vi "SEK2020v1SubVIAndarReto.vi"(1 "NXT/EV3":T1) -> (8 "NXT/EV3 2":T1)   [LabVIEW 2016]
uses:
  <vilib>/NXT/Subs/LVHSConnector.ctl
  <vilib>/NXT/LegoClasses/BrickReference/BrickReference.lvclass
  <vilib>/NXT/Block Support/NXT_InputPort.ctl
  <vilib>/NXT/Block Support/NXT_OutputPort.ctl
  <vilib>/NXT/Dual Mode Library/Sensors/EV3_Gyro_Angle.vi
  <vilib>/NXT/Dual Mode Library/Waits/Wait_Num.vi
  <vilib>/NXT/NXTIO Xnodes/NXTIONodeSubVIs/NXTMoveMotors.vi
  <vilib>/NXT/NXTIO Xnodes/AddressXNode/NXTIOAddress.xnode
  <vilib>/NXT/NXTIO Xnodes/NXTIOXNode/NXTIO.xnode
panel:
  in  "Kd":sgl
  in  "Ki":sgl
  in  "Kp":sgl=2.0
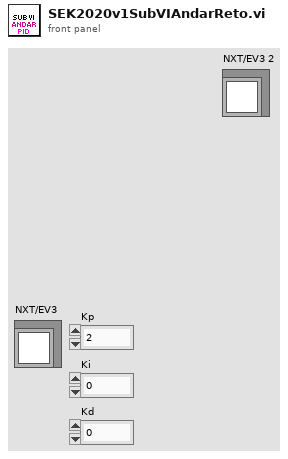
[diagram p1: front panel]
types:
  T1 = typedef "LVHSConnector.ctl" = refnum<class "BrickReference.lvclass">
  T2 = typedef "NXT_InputPort.ctl" = u32
  T3 = typedef "NXT_OutputPort.ctl" = u8
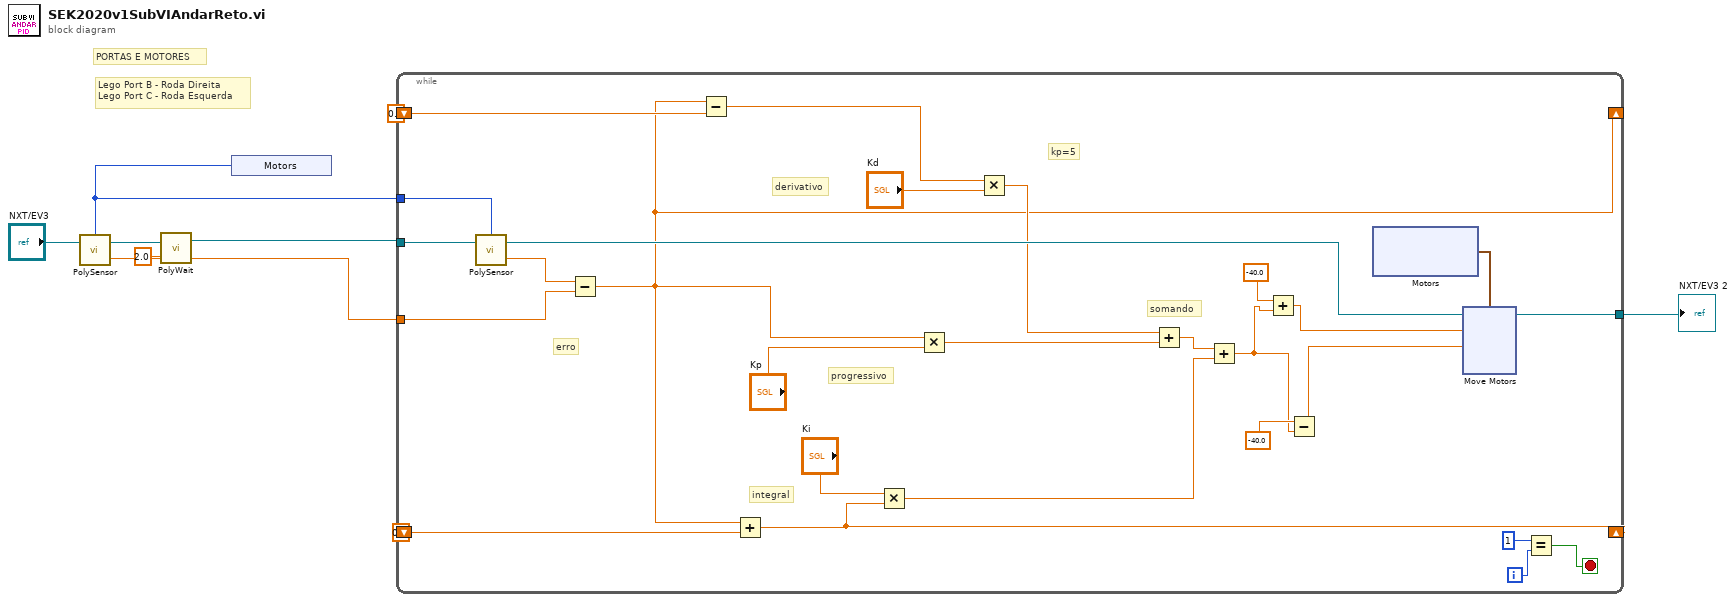
[diagram p0: block diagram]
diagram:
  # "Lego Port B - Roda Direita\nLego Port C - Roda Esquerda"
  # "PORTAS E MOTORES"
  n1 = xnode "Motors"() -> ("Sensor"=w6:T2)
  n2 = call-poly <vilib>:"PolySensor.vi"("NXT/EV3"="NXT/EV3", "Port (Port 1)"=w6) -> ("Degrees"=w5:sgl, "NXT/EV3"=w3:T1)  [unwired: 1 in]
  n3 = call-poly <vilib>:"PolyWait.vi"("Time (1 sec)"=sgl 2.0, "NXT/EV3"=w3) -> ("NXT/EV3"=w2:T1)  [unwired: 2 in]
  n4 = while {
    tunnel: w2 -> [w36]
    shift-right: [w28] -> _
    shift-left: sgl 0.0 -> [w30]
    shift-right: [w23] -> _
    shift-left: sgl 0.0 -> [w25]
    tunnel: w6 -> [w20]
    tunnel: w5 -> [w19]
    tunnel: [w13] -> w4
    i -> [w12]
    stop <- w10 stop-if-true
    # "kp=5"
    # "somando"
    # "erro"
    # "progressivo"
    # "integral"
    # "derivativo"
    n5 = call-poly <vilib>:"PolySensor.vi"("NXT/EV3"=w36, "Port (Port 1)"=w20) -> ("Degrees"=w24:sgl, "NXT/EV3"=w31:T1)  [unwired: 1 in]
    n6 = Subtract(x=w24, y=w19) -> (x-y=w23:sgl)
    n7 = Subtract(x=w23, y=w25) -> (x-y=w21:sgl)
    n8 = Add(x=w23, y=w30) -> (x+y=w28:sgl)
    n9 = Multiply(x="Ki", y=w28) -> (x*y=w27:sgl)
    n10 = Multiply(x=w23, y="Kp") -> (x*y=w33:sgl)
    n11 = Multiply(x=w21, y="Kd") -> (x*y=w26:sgl)
    n12 = Add(x=w26, y=w33) -> (x+y=w32:sgl)
    n13 = Add(x=w32, y=w27) -> (x+y=w14:sgl)
    n14 = Add(x=sgl -40.0, y=w14) -> (x+y=w17:sgl)
    n15 = Subtract(x=sgl -40.0, y=w14) -> (x-y=w16:sgl)
    n16 = xnode "Motors"() -> ("Motor"=w35:cluster{"Port":T3, "Port":T3})
    n17 = xnode "Move Motors"("Power/Speed 2"=w16, "Power/Speed 1"=w17, "Motors"=w35, "NXT/EV3"=w31) -> ("NXT/EV3"=w13:T1)
    n18 = Equal?(x=1, y=w12) -> (x = y?=w10:bool)
  }
  "NXT/EV3 2" <- w4
